vi "MoveXYZ.vi"(1 "X final height":dbl, 3 "Y final height":dbl, 5 "Z final height":dbl, 8 "Set X":bool, 9 "V final":dbl, 10 "Set Y":bool, 11 "Scan Rate (um/s)":dbl=15.0, 12 "Set Z":bool, 13 "Scan Rate (V/s) 2":dbl=15.0, 14 "Set Voltage":bool) -> ()   [LabVIEW 2023]
uses:
  TypeDefs/Settings.ctl
  TypeDefs/WayPointCluster.ctl
panel:
  in  "WayPointCluster":T1
  in  "SettingsCluster":T2={"Sample Rate (us)"=1, "Samples Per Data Point (int, power of 2)"=1000, "DistanceToBulk (um)"=-1.0, "HoldTimeScaler"=0, "SaveData"=FALSE, "DistanceToBulk (um) 2"=-1.0, "DistanceToBulk (um) 3"=-1.0}
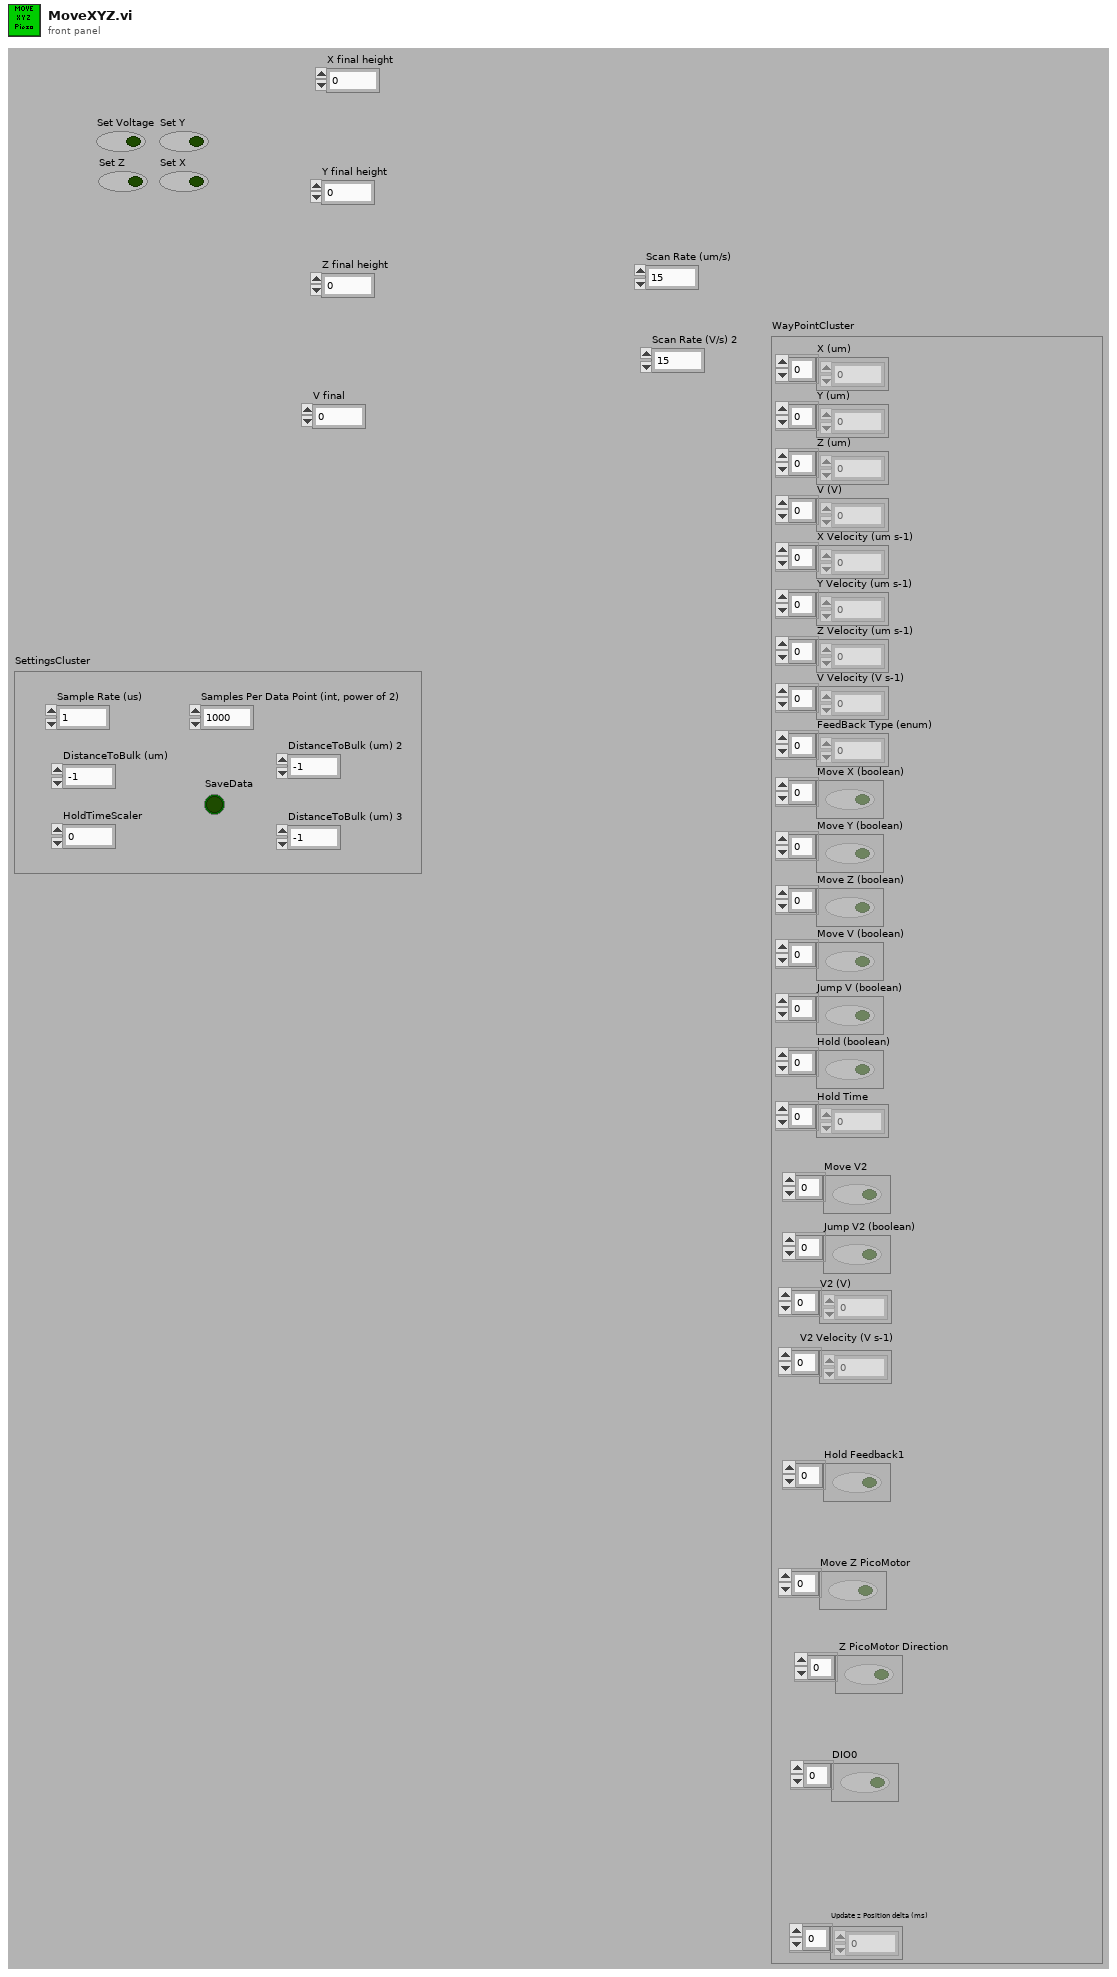
[diagram p1: front panel]
types:
  T1 = typedef "WayPointCluster.ctl" = cluster{"X (um)":dbl[], "Y (um)":dbl[], "Z (um)":dbl[], "V (V)":dbl[], "X Velocity (um s-1)":dbl[], "Y Velocity (um s-1)":dbl[], "Z Velocity (um s-1)":dbl[], "V Velocity (V s-1)":dbl[], "FeedBack Type (enum)":u16[], "Move X (boolean)":bool[], "Move Y (boolean)":bool[], "Move Z (boolean)":bool[], "Move V (boolean)":bool[], "Jump V (boolean)":bool[], "Hold (boolean)":bool[], "Hold Time":u32[], "V2 (V)":dbl[], "Move V2":bool[], "V2 Velocity (V s-1)":dbl[], "Jump V2 (boolean)":bool[], "Update z Position delta (ms)":i16[], "Hold Feedback1":bool[], "Move Z PicoMotor":bool[], " Z PicoMotor Direction":bool[], "DIO0":bool[]}
  T2 = typedef "Settings.ctl" = cluster{"Sample Rate (us)":u32, "Samples Per Data Point (int, power of 2)":i16, "DistanceToBulk (um)":dbl, "HoldTimeScaler":u64, "SaveData":bool, "DistanceToBulk (um) 2":dbl, "DistanceToBulk (um) 3":dbl}
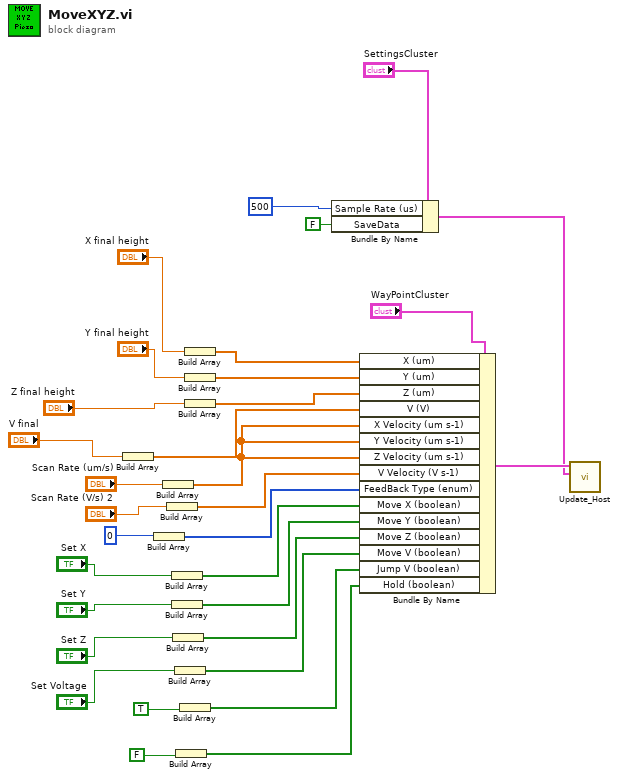
[diagram p0: block diagram]
diagram:
  n1 = Build Array("V final") -> (w25:dbl[])
  n2 = Build Array(u16 0 ("Update Position Loop Wait Time (us)")) -> (w18:u16[])
  n3 = Build Array("Scan Rate (um/s)") -> (w23:dbl[])
  n4 = Build Array("Scan Rate (V/s) 2") -> (w24:dbl[])
  n5 = Build Array("Set X") -> (w15:bool[])
  n6 = Build Array("Set Y") -> (w13:bool[])
  n7 = Build Array("Set Z") -> (w11:bool[])
  n8 = Build Array("Set Voltage") -> (w9:bool[])
  n9 = Build Array(FALSE ("Set Voltage")) -> (w4:bool[])
  n10 = Build Array(TRUE ("Set Voltage")) -> (w7:bool[])
  n11 = Build Array("X final height") -> (w28:dbl[])
  n12 = Build Array("Y final height") -> (w27:dbl[])
  n13 = Build Array("Z final height") -> (w26:dbl[])
  n14 = Bundle By Name(cluster="SettingsCluster", "Sample Rate (us)"=u32 500 ("Buffer and feedback Loop Wait Time (us)"), "SaveData"=FALSE) -> (w8:T2)
  n15 = Bundle By Name(cluster="WayPointCluster", "X (um)"=w28, "Y (um)"=w27, "Z (um)"=w26, "V (V)"=w25, "X Velocity (um s-1)"=w23, "Y Velocity (um s-1)"=w23, "Z Velocity (um s-1)"=w23, "V Velocity (V s-1)"=w24, "FeedBack Type (enum)"=w18, "Move X (boolean)"=w15, "Move Y (boolean)"=w13, "Move Z (boolean)"=w11, "Move V (boolean)"=w9, "Jump V (boolean)"=w7, "Hold (boolean)"=w4) -> (w17:T1)
  n16 = call "Update_Host.vi"("SettingsCluster"=w8, "WayPointCluster"=w17) -> ()  [unwired: 8 in]
